vi "FSM.vi"() -> ()   [LabVIEW 2016]
doc: "Use this template to build a simple state machine design pattern. Each state executes code and determines which state to transition to."
uses:
  controls/State.ctl
panel:
  out "Long":bool
  in  "stop":bool
  in  "input1":bool
  in  "input 0":bool
  out "Select Sentence":bool
  out "Word Outputs":string[](array[string])=["", "", "", "", "", "", "", "h", "i", "j", "k", "l", "m", "n", "o", "p", "q", "r", "s", "t", "u", "v", "w", "x", "y", "z"]
  out "Length counter":i32
  out "Input RMS":dbl
  out "Slide":T1 scale=0.0..100.0
  in  "Dictionary Path":path
  out "DIGITS":string
  out "Letters Output":string
  in  "sentence2":string
  in  "sentence1":string
  in  "停止按钮":bool
  out "one":bool
  out "zero":bool
  in  "RMS threshold":dbl
  in  "Length threshold":i32=20
  in  "Input Gain":dbl
  out "Frequency response":dynamicdata(graph)
  out "Short":bool
  in  "Input TEST":dbl(slide) scale=0.0..10.0
  out "数组":string[](array[string])
  out "testforlin":string
  out "三位数":i32
  out "count digit":i32
  out "check code":bool
  out "Digits 2":bool[](array[boolean])
  out "index word mode":dbl
  out "add 0 （word mode）":bool
  out "counter2":dbl
  out "counter":dbl
  out "word index":dbl
  out "compare word":string
  out "Final Output":string
  out "instructions":string[](array[string])=["Hello", "Run", "Phone", "Cat", "Speak", "Mango", "Late", "EMG", "Volleyball", "Sing", "Over", "Maybe", "After", "Banana", "Love", "Sleep", "Too", "Hope", "Tomorrow", "Smile"]
  out "Last selected letter":string
  out "letters output (array)":string[](array[string])
  out "Current letter index":dbl
  out "Digits":bool[](array[boolean])
  out "Current digit index":dbl
  out "letter database":string[](array[string])=["Hello", "Run", "Phone", "Cat", "Speak", "Mango", "Late", "EMG", "Volleyball", "Sing", "Over", "Maybe", "After", "Banana", "Love", "Sleep", "Too", "Hope", "Tomorrow", "Smile"]
  out "Current state":T2=enum."Count digits"
  in  "Exit":bool
  # "Instruction Code:"
  # "Suggesting\nList"
  # "10000    p\n10001    q\n10010    r\n10011    s\n10100    t\n10101    u\n10110    v\n10111    w\n11000    x\n11001    y\n11010    z\n11011    clear letter\n11100    clear sentence\n\n11101    enter sentence 1\n\n\n11110    enter sentence 2\n\n11111    select word"
  # "00000    enter\n00001    a\n00010    b\n00011    c\n00100    d\n00101    e\n00110    f\n00111    g\n01000    h\n01001    i\n01010    j\n01011    k\n01100    l\n01101    m\n01110    n\n01111    o"
  # "TESTING"
  # "Input Parameters"
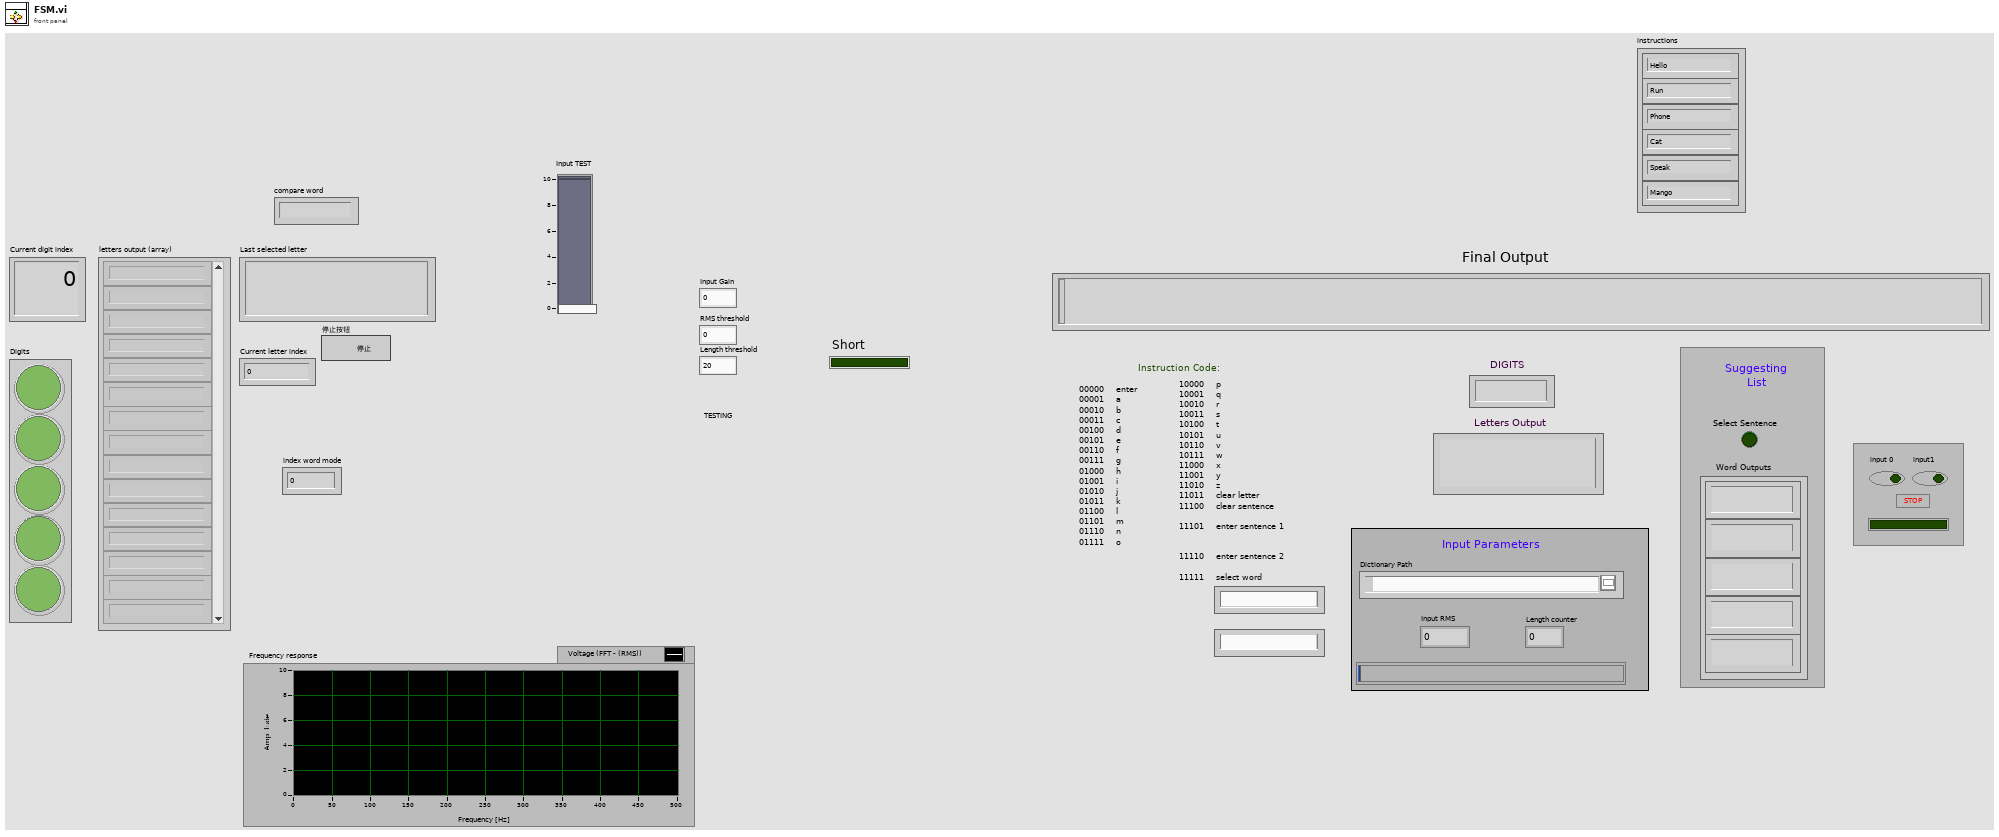
[diagram p1: front panel]
types:
  T1 = typedef "控件 1.ctl" = u8
  T2 = typedef "State.ctl" = enum16{"check code for word", "count digit for word", "add 1 word", "add 0 word", "pick word", "enter sentence3", "enter sentence2", "enter sentence1", "clear sentence", "enter word", "clear all", "check code", "Count digits", "Input signal", "Add digit 0", "Add digit 1", "Select word", "Reset digits", "Delete word", "Exit"}
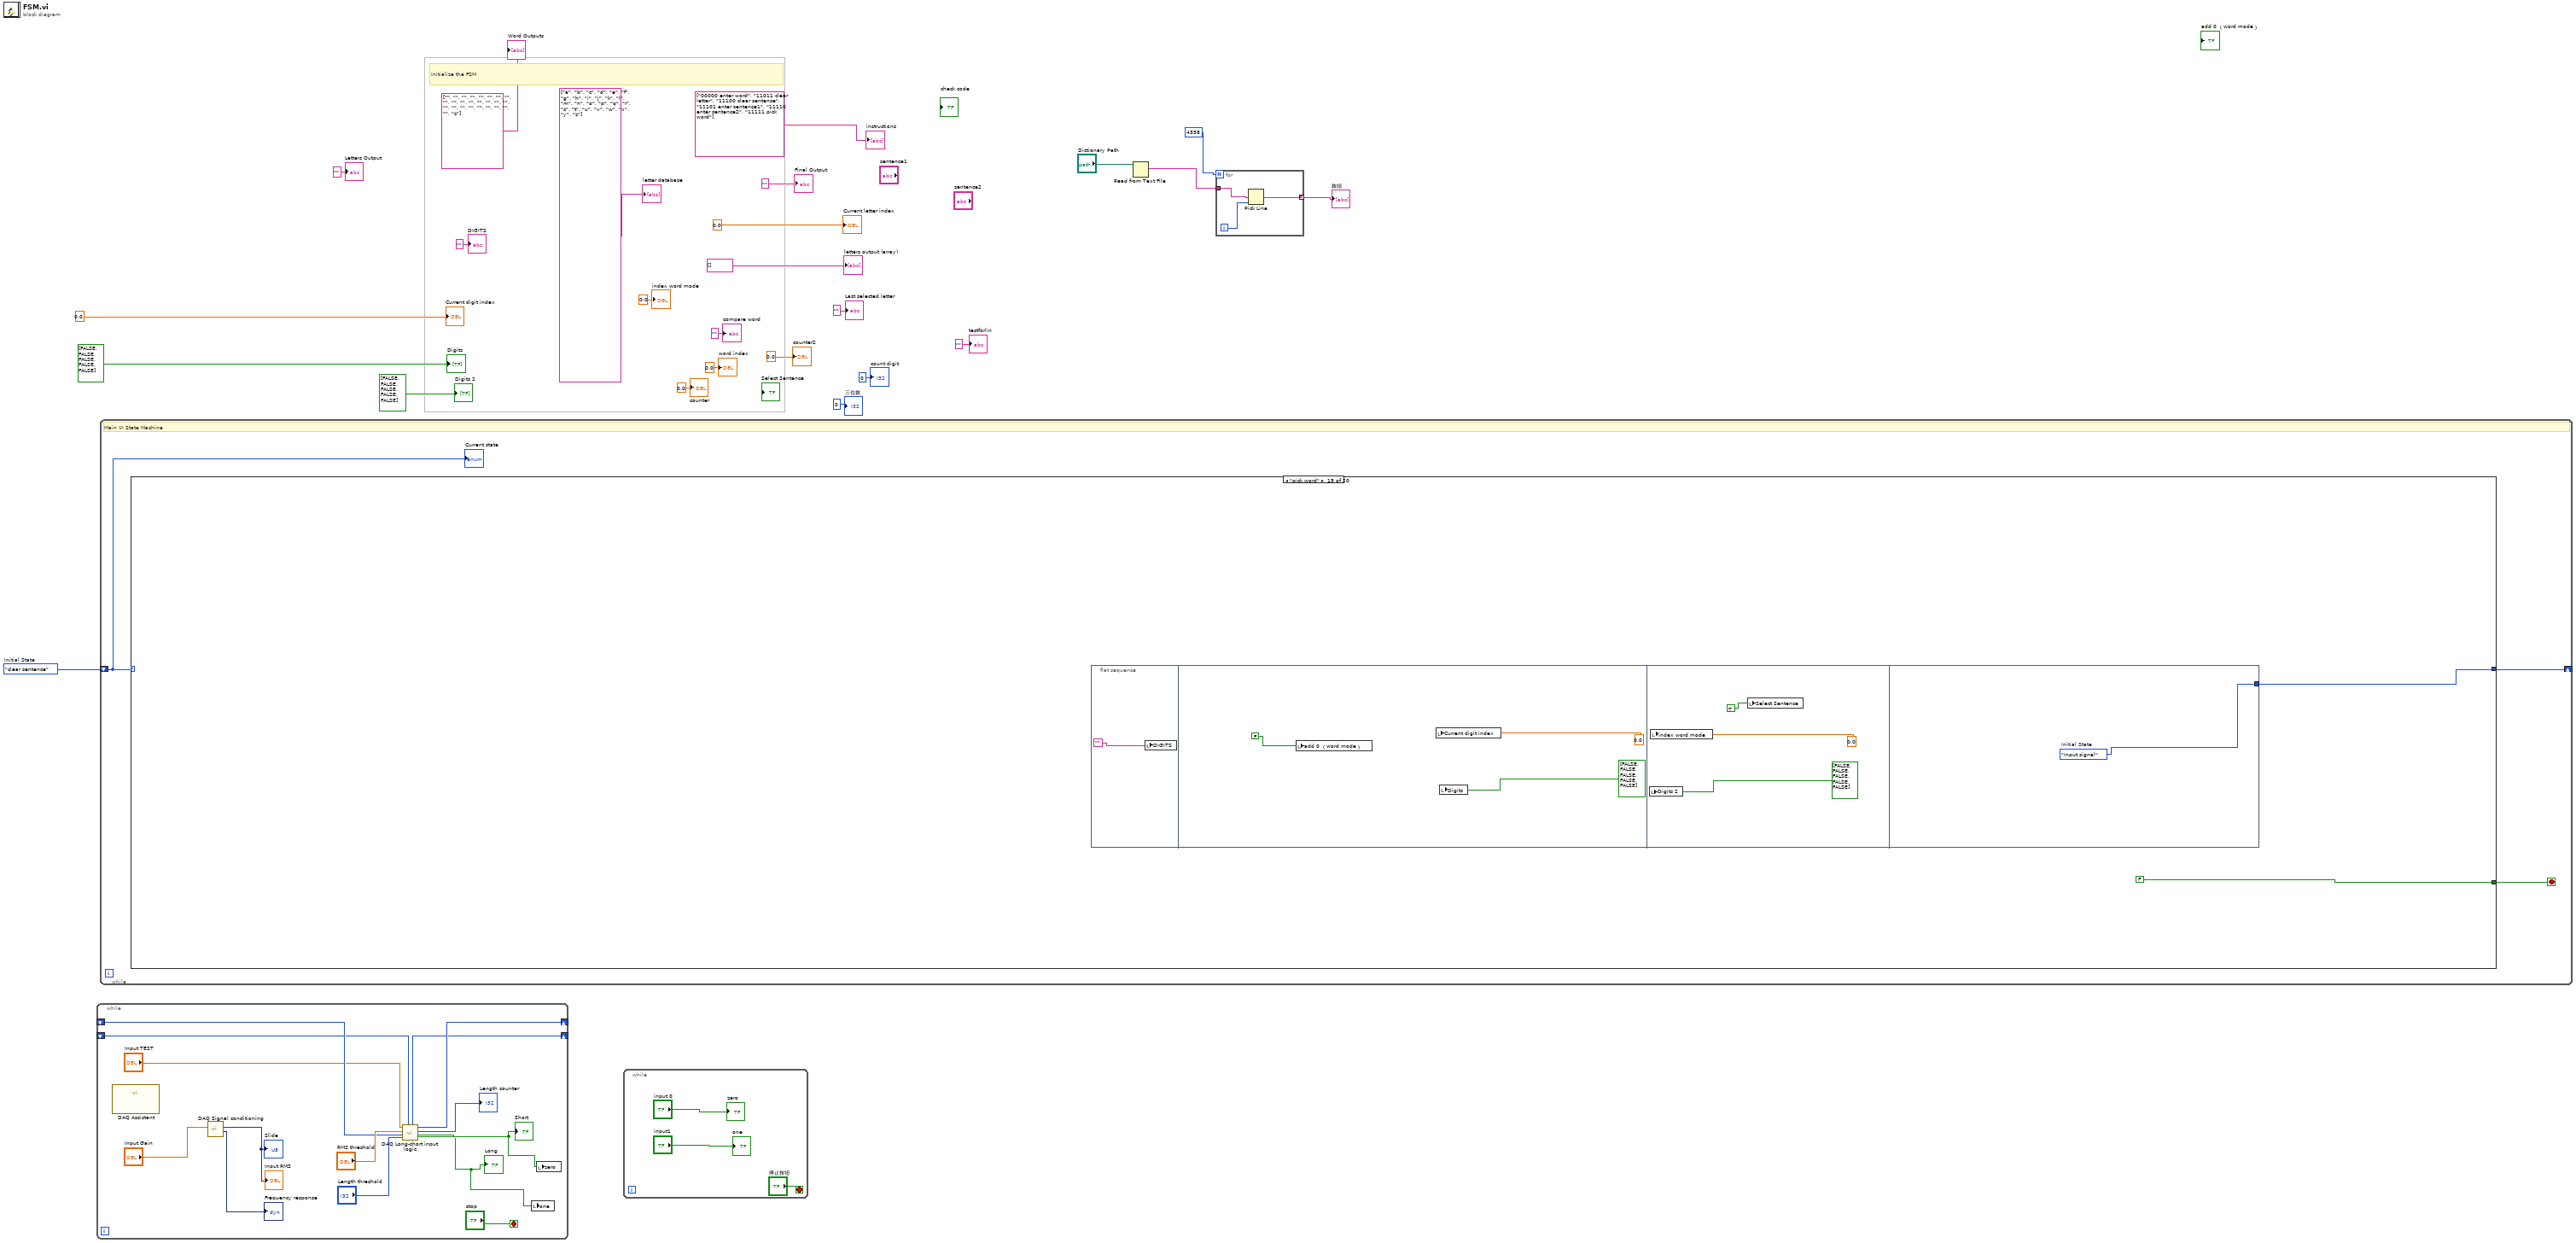
[diagram p0: block diagram]
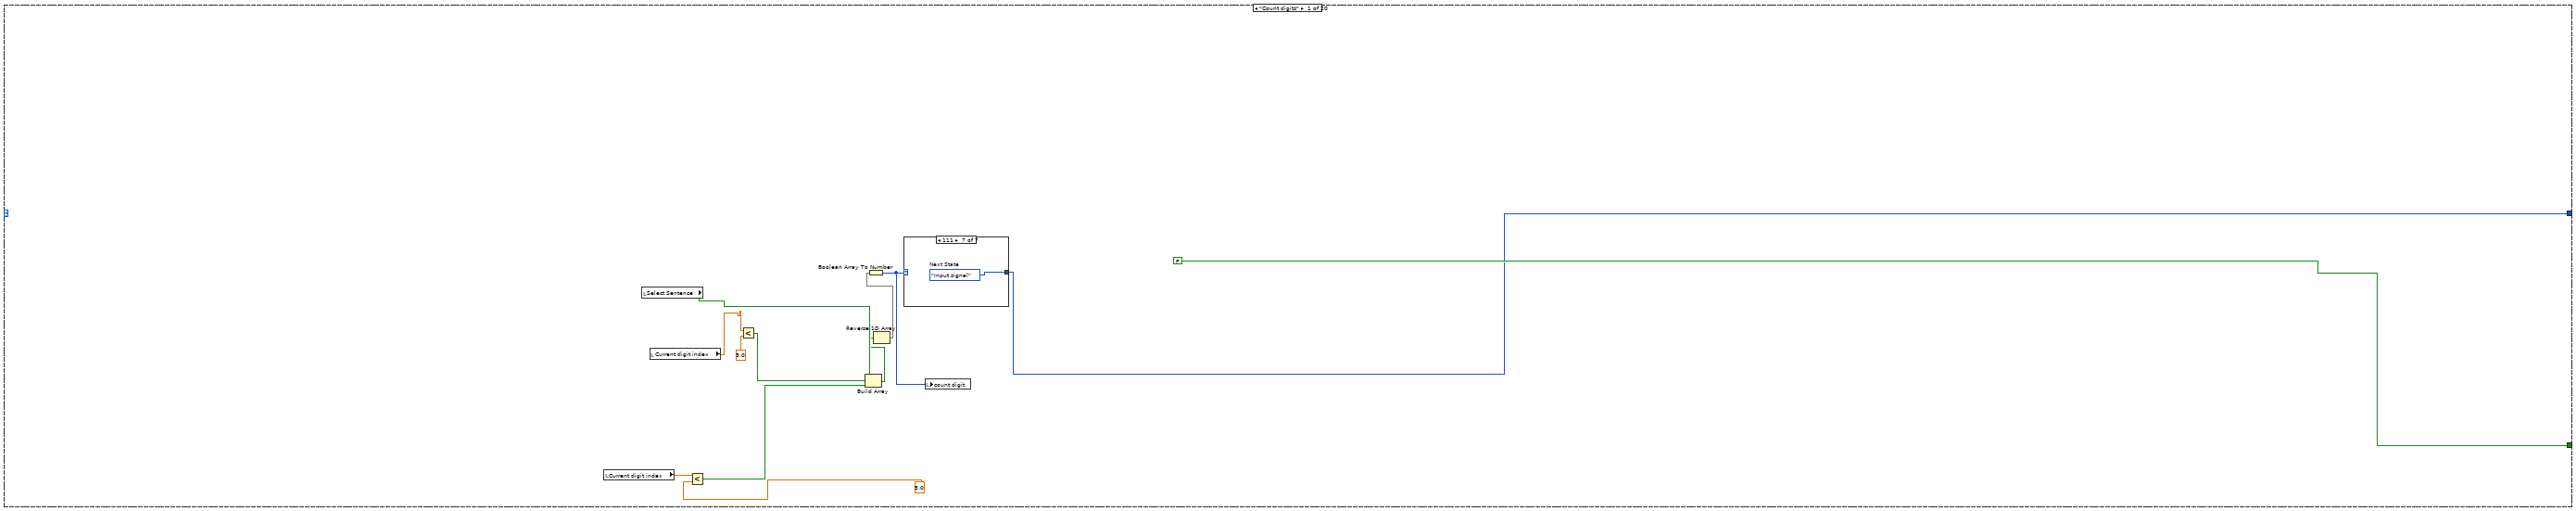
[diagram p2: hidden frame]
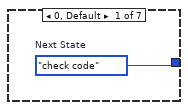
[diagram p3: hidden frame]
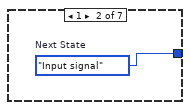
[diagram p4: hidden frame]
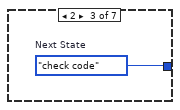
[diagram p5: hidden frame]
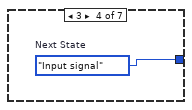
[diagram p6: hidden frame]
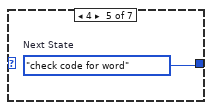
[diagram p7: hidden frame]
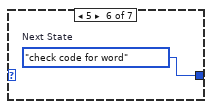
[diagram p8: hidden frame]
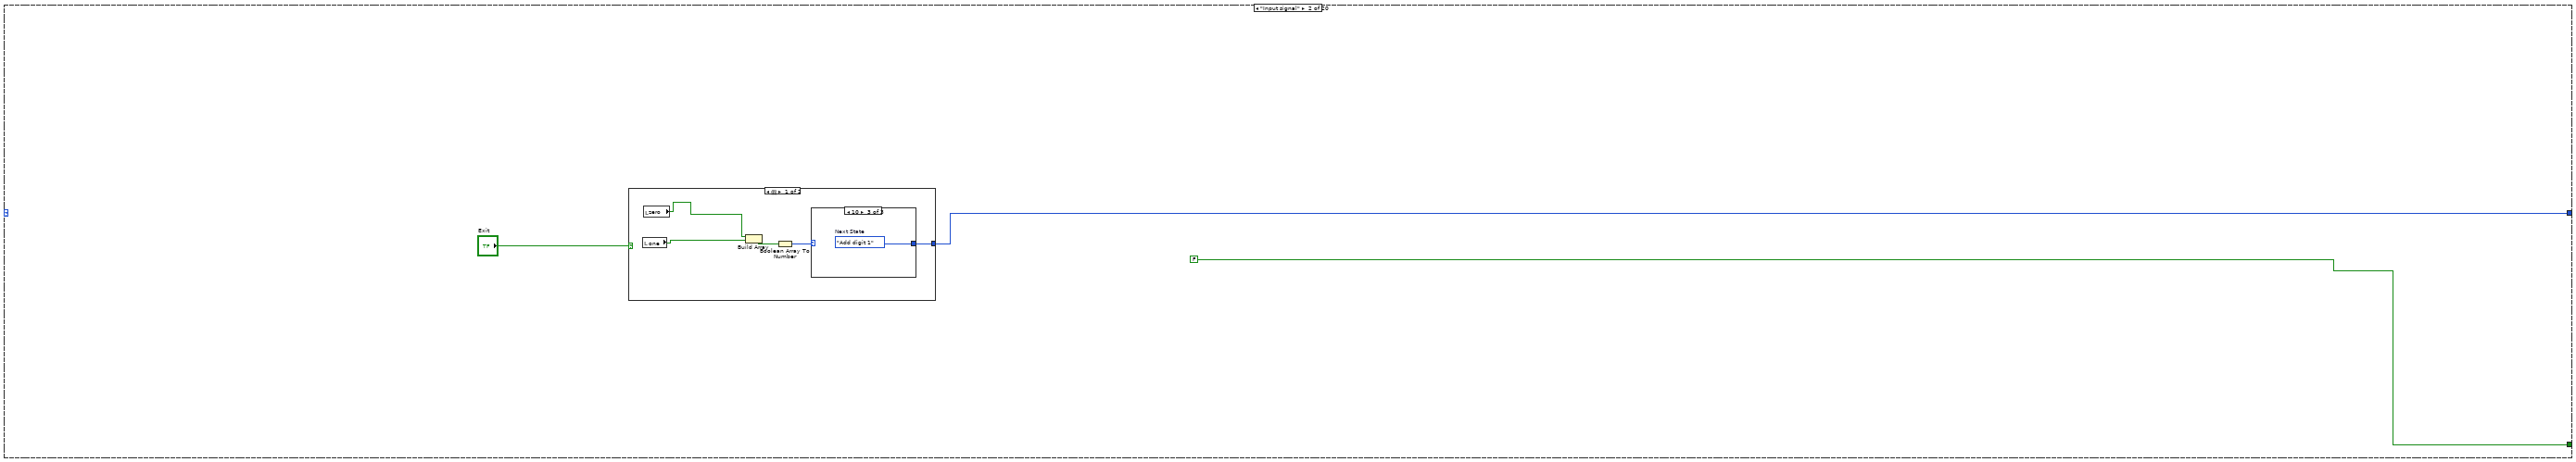
[diagram p9: hidden frame]
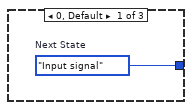
[diagram p10: hidden frame]
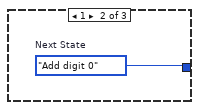
[diagram p11: hidden frame]
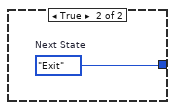
[diagram p12: hidden frame]
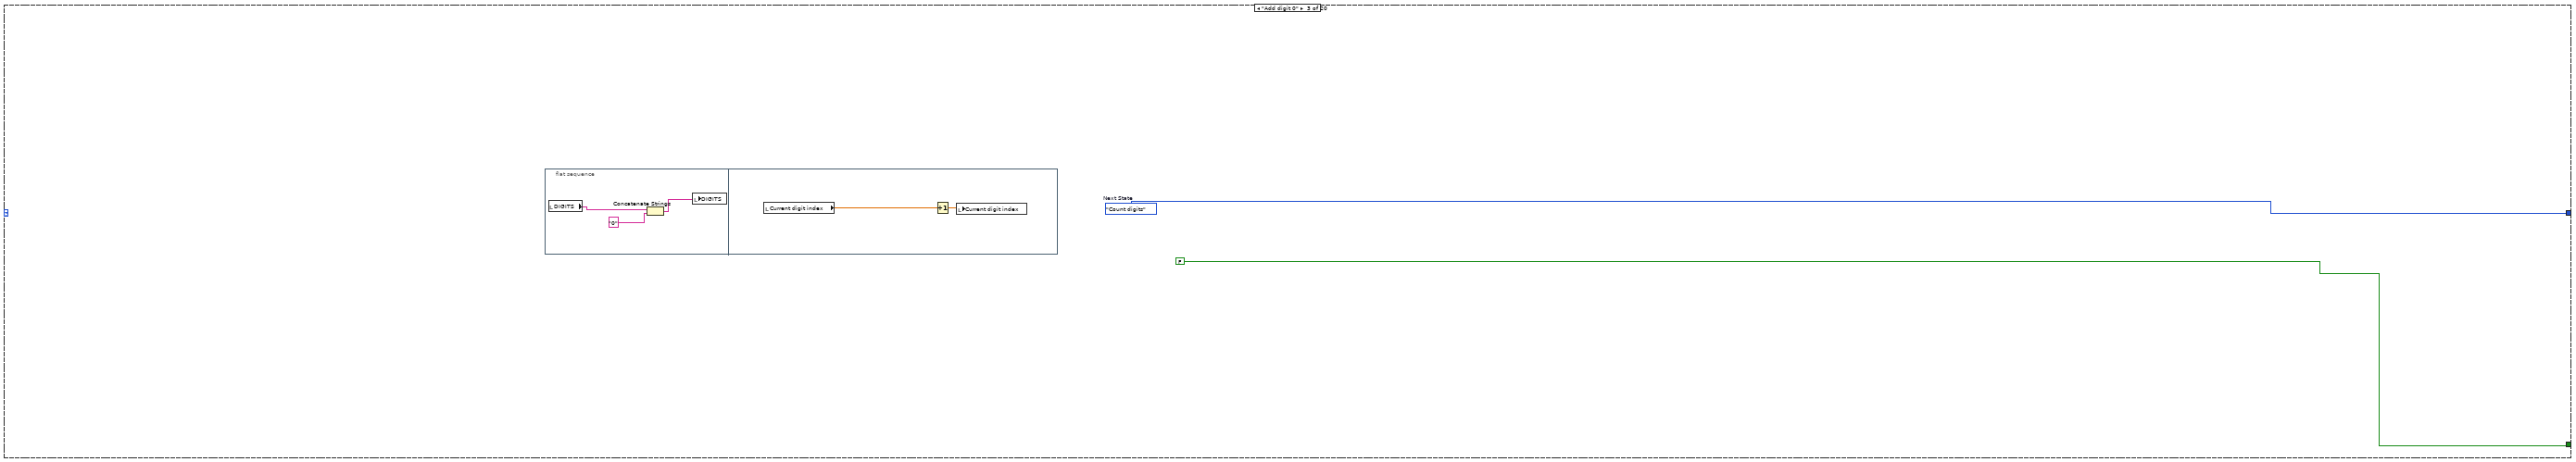
[diagram p13: hidden frame]
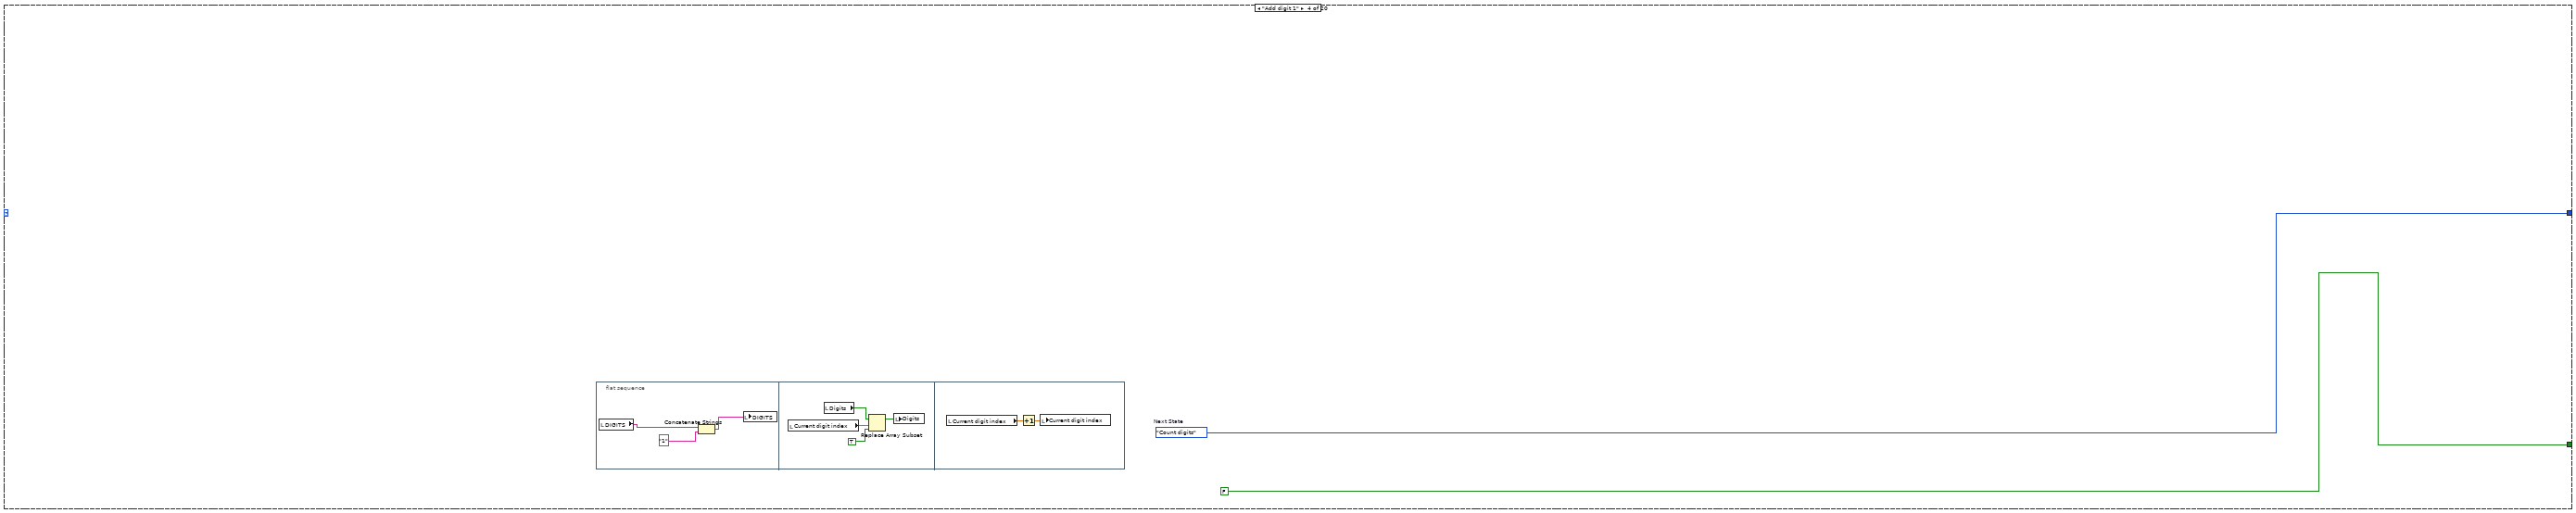
[diagram p14: hidden frame]
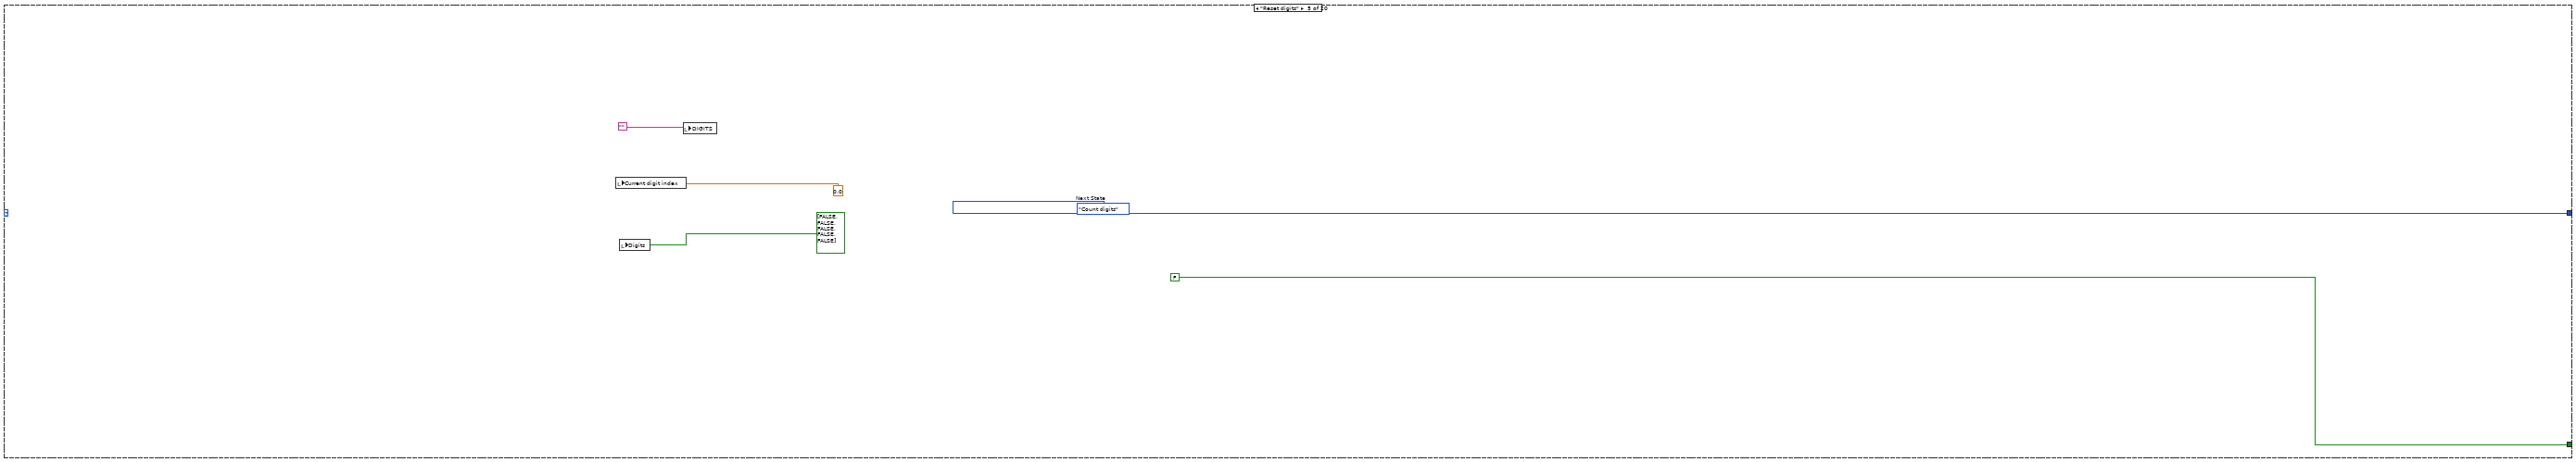
[diagram p15: hidden frame]
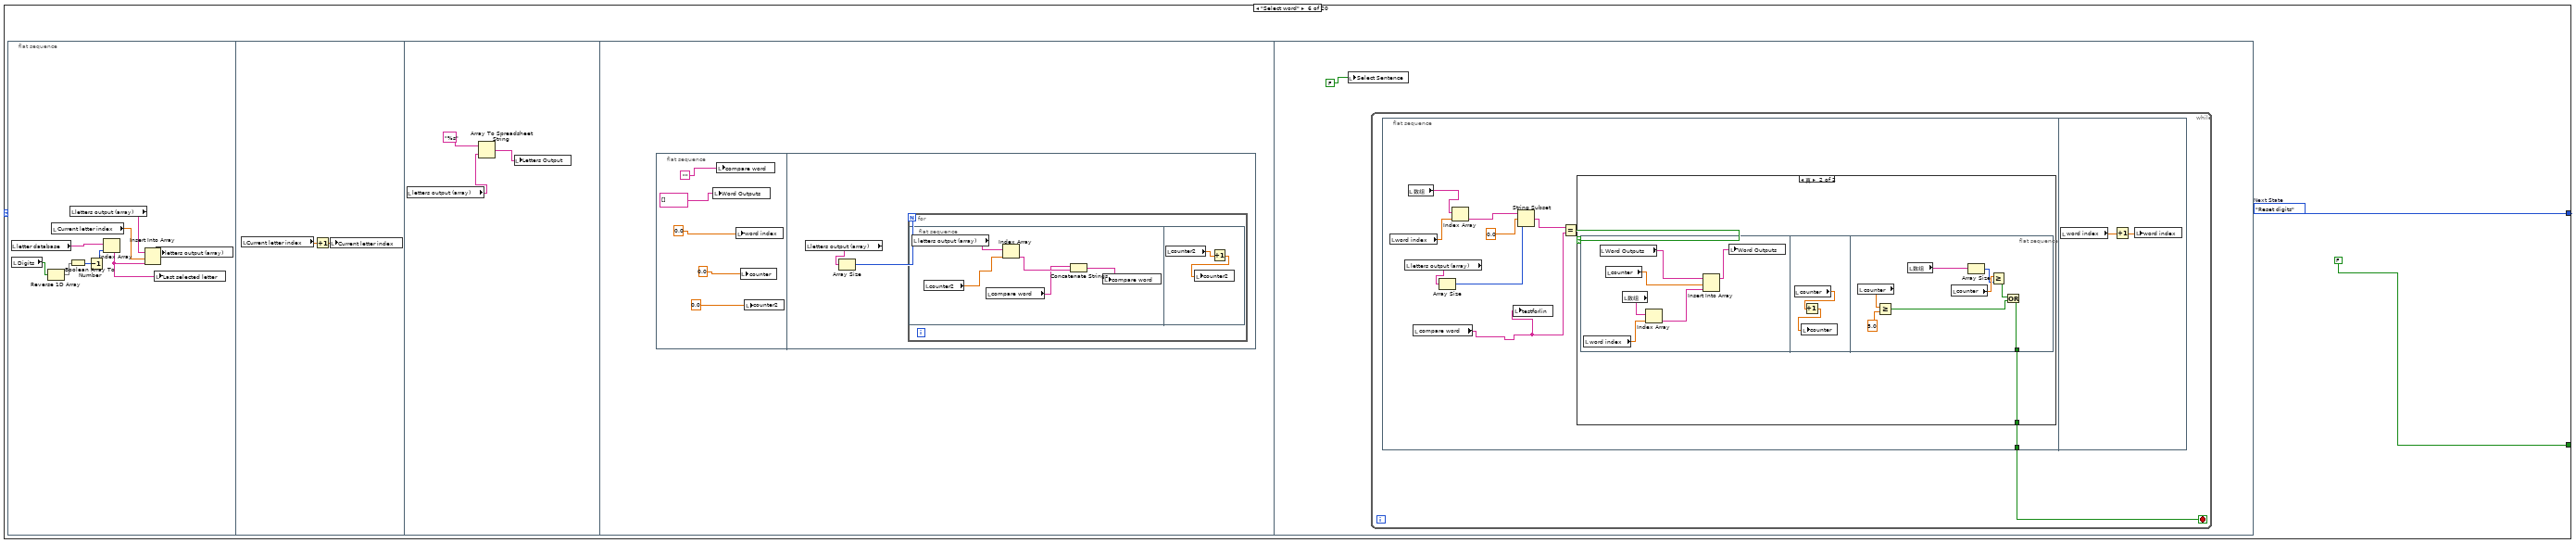
[diagram p16: hidden frame]
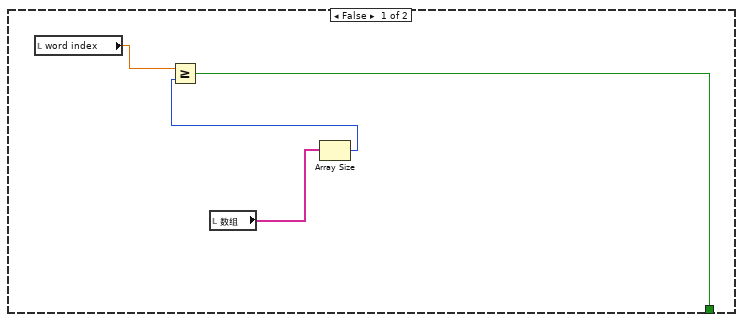
[diagram p17: hidden frame]
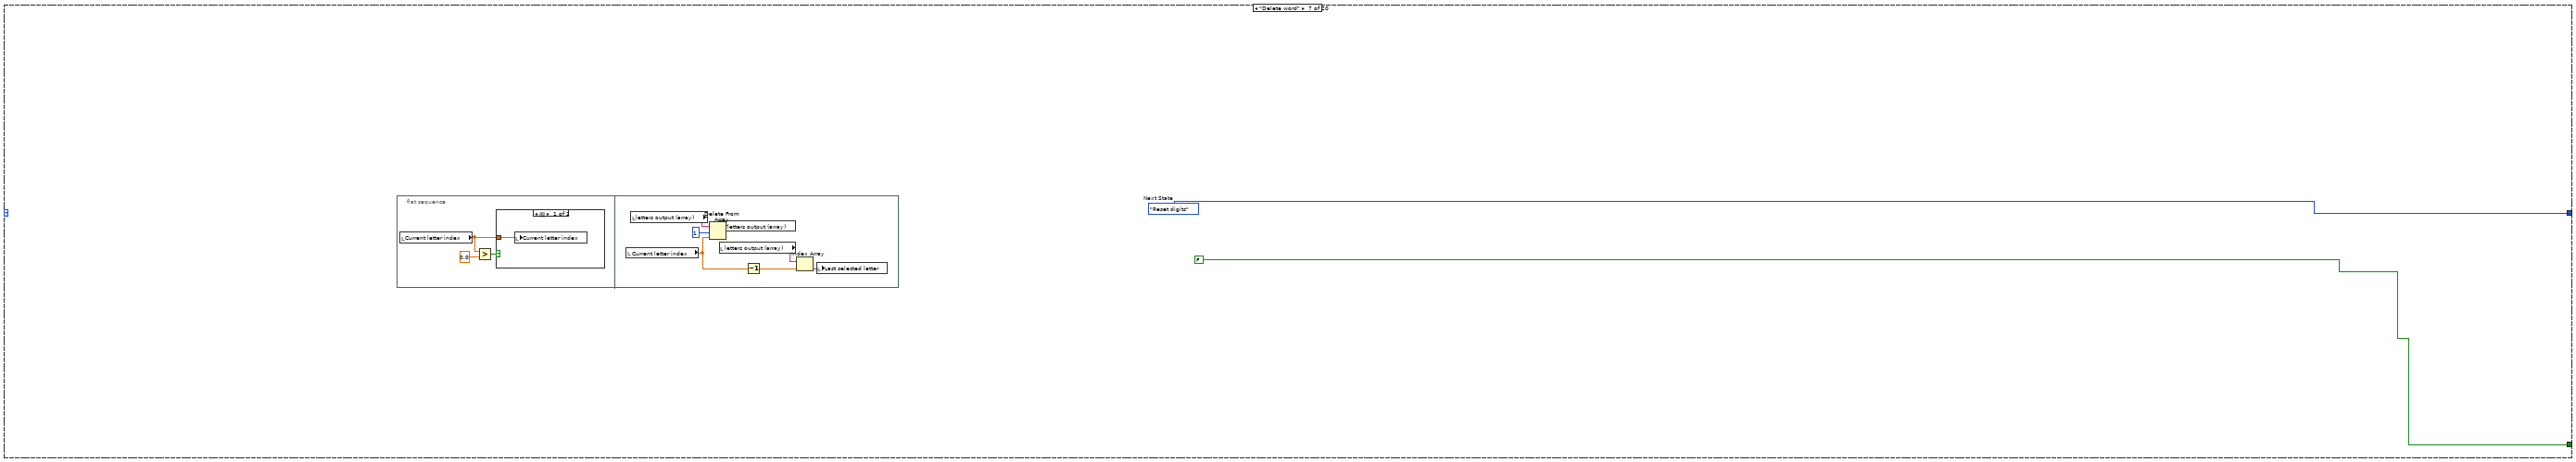
[diagram p18: hidden frame]
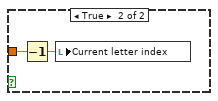
[diagram p19: hidden frame]
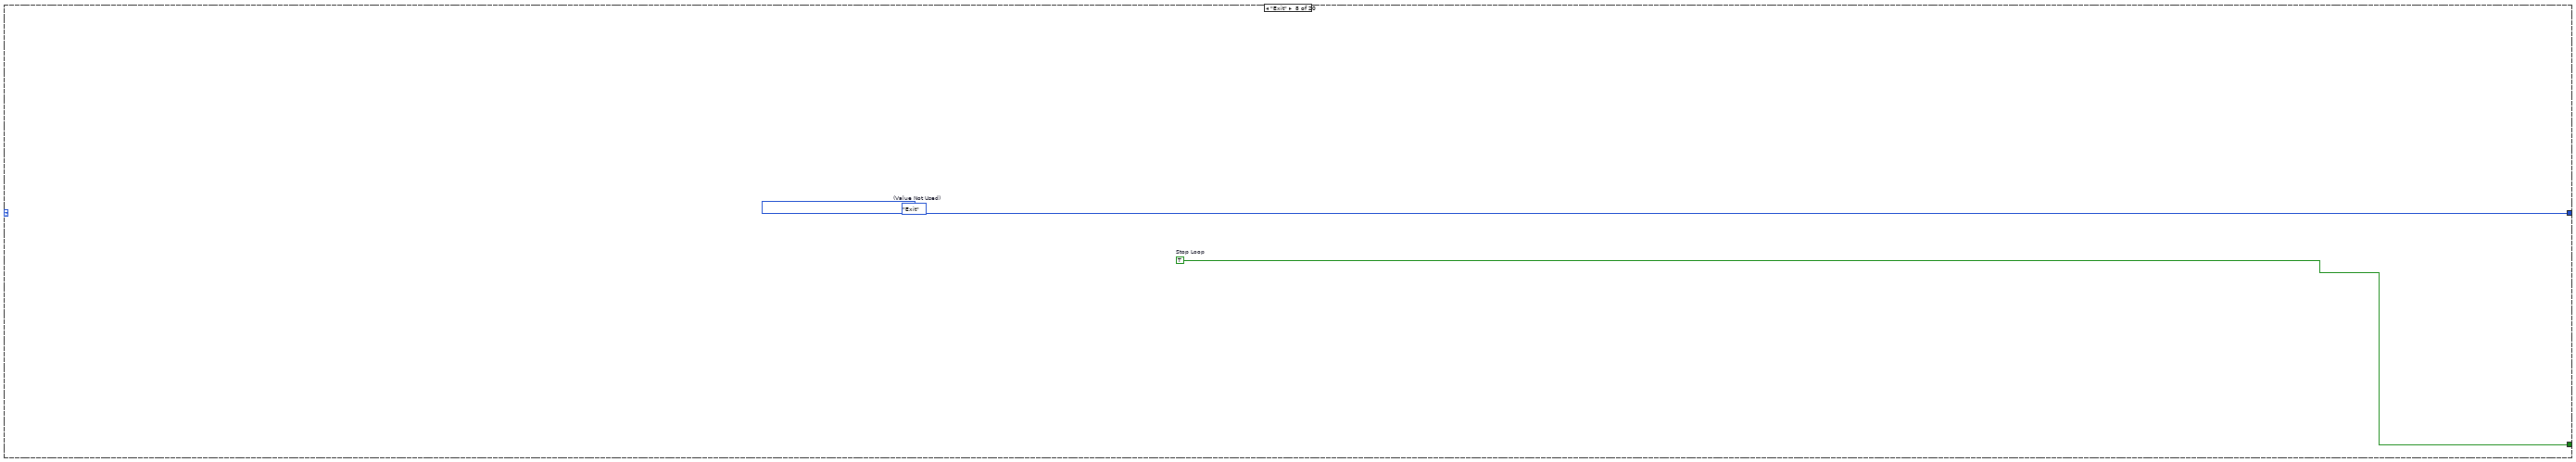
[diagram p20: hidden frame]
diagram:
  w25 = State."clear sentence"  # Initial State
  # "Initialize the FSM"
  n1 = while {
    shift-right: [w37] -> _
    shift-left: _ -> [w36]
    shift-right: [w34] -> _
    shift-left: _ -> [w35]
    stop <- "stop" stop-if-true
    n2 = call "DAQ Assistant"() -> ()  [unwired: 12 in]
    n3 = call "DAQ Signal conditioning.vi"("Gain"="Input Gain") -> ("FFT - (RMS)"=→"Frequency response":dynamicdata, "Dynamic Data"=→"Input RMS" →"Slide":dynamicdata)  [unwired: 9 in]
    n4 = call "DAQ Long-short input logic.vi"("Signal Length"="Length threshold", "Numeric in"=w35, "Numeric 3"=w36, "Threshold"="RMS threshold", "data"="Input TEST") -> ("Boolean"=w27:bool, "x+y"=→"Length counter":i32, "Numeric 4"=w37:i32, "Boolean 2"=w26:bool, "Numeric out"=w34:i32)  [unwired: 2 in]
    "Short" <- w27
    "Long" <- w26
    n5 = local write "one"(w26) -> ()
    n6 = local write "zero"(w27) -> ()
  }
  n7 = while {
    shift-right: [w41] -> _
    shift-left: w25 -> [w42]
    stop <- w40 stop-if-true
    # "Main VI State Machine"
    n8 = case "条件结构" shown="\"pick word\"" w42 {
      tunnel: [w49 w64 w75 w82 w96 w98 w163 w178 w184 w202 w212 w227 w231 w236 w240 w244 w249 w257 w265 w275] -> w41
      tunnel: [FALSE FALSE FALSE FALSE FALSE FALSE ("Stop Loop?") FALSE ("Stop Loop?") w177 FALSE FALSE FALSE FALSE FALSE FALSE FALSE FALSE FALSE FALSE FALSE FALSE] -> w40
      frame "Count digits" {
        n9 = local read "Current digit index"() -> (w52:dbl)
        n10 = local read "Select Sentence"() -> (w46:bool)
        n11 = local read "Current digit index"() -> (w51:dbl)
        n12 = Less?(x=w52, y=5.0) -> (x < y?=w45:bool)
        n13 = Less?(x=w51, y=3.0) -> (x < y?=w48:bool)
        n14 = Build Array(w46, w48, w45) -> (w43:bool[])
        n15 = Reverse 1D Array(array=w43) -> (reversed array=w44:bool[])
        n16 = Boolean Array To Number(Boolean array=w44) -> (number=w47:u32)
        n17 = case shown="111" w47 {
          tunnel: [w55 w56 w57 w58 w59 w60 w61] -> w49
          frame 0, Default {
            w55 = State."check code"  # Next State
          }
          frame 1 {
            w56 = State."Input signal"  # Next State
          }
          frame 2 {
            w57 = State."check code"  # Next State
          }
          frame 3 {
            w58 = State."Input signal"  # Next State
          }
          frame 4 {
            w59 = State."check code for word"  # Next State
          }
          frame 5 {
            w60 = State."check code for word"  # Next State
          }
          frame 7 {
            w61 = State."Input signal"  # Next State
          }
        }
        n18 = local write "count digit"(w47) -> ()
      }
      frame "Input signal" {
        n19 = case shown="假" "Exit" {
          tunnel: [w67 w73] -> w64
          frame False {
            n20 = local read "one"() -> (w65:bool)
            n21 = local read "zero"() -> (w66:bool)
            n22 = Build Array(w66, w65) -> (w69:bool[])
            n23 = Boolean Array To Number(Boolean array=w69) -> (number=w68:u32)
            n24 = case shown="10" w68 {
              tunnel: [w70 w71 w72] -> w67
              frame 0, Default {
                w70 = State."Input signal"  # Next State
              }
              frame 1 {
                w71 = State."Add digit 0"  # Next State
              }
              frame 2 {
                w72 = State."Add digit 1"  # Next State
              }
            }
          }
          frame True {
            w73 = State."Exit"  # Next State
          }
        }
      }
      frame "Add digit 0" {
        w75 = State."Count digits"  # Next State
        n25 = flat-sequence {
          frame #0 {
            n26 = local read "DIGITS"() -> (w76:string)
            n27 = Concatenate Strings(w76, "0") -> (w78:string)
            n28 = local write "DIGITS"(w78) -> ()
          }
          frame #1 {
            n29 = local read "Current digit index"() -> (w80:dbl)
            n30 = Increment(x=w80) -> (x+1=w79:dbl)
            n31 = local write "Current digit index"(w79) -> ()
          }
        }
      }
      frame "Add digit 1" {
        w82 = State."Count digits"  # Next State
        n32 = flat-sequence {
          frame #0 {
            n33 = local read "DIGITS"() -> (w85:string)
            n34 = Concatenate Strings(w85, "1") -> (w83:string)
            n35 = local write "DIGITS"(w83) -> ()
          }
          frame #1 {
            n36 = local read "Current digit index"() -> (w89:dbl)
            n37 = local read "Digits"() -> (w87:bool[])
            n38 = Replace Array Subset(array=w87, new element=TRUE, index=w89) -> (w86:bool[])
            n39 = local write "Digits"(w86) -> ()
          }
          frame #2 {
            n40 = local read "Current digit index"() -> (w91:dbl)
            n41 = Increment(x=w91) -> (x+1=w90:dbl)
            n42 = local write "Current digit index"(w90) -> ()
          }
        }
      }
      frame "Reset digits" {
        w96 = State."Count digits"  # Next State
        n43 = local write "Current digit index"(0.0 ("Current digit index")) -> ()
        n44 = local write "Digits"(bool[] [FALSE, FALSE, FALSE, FALSE, FALSE]) -> ()
        n45 = local write "DIGITS"("") -> ()
      }
      frame "Select word" {
        w98 = State."Reset digits"  # Next State
        # "User State 1 - Replace this state with functionality for your own application."
        n46 = flat-sequence {
          frame #0 {
            n47 = local read "letter database"() -> (w104:string[])
            n48 = local read "Digits"() -> (w102:bool[])
            n49 = Reverse 1D Array(array=w102) -> (reversed array=w101:bool[])
            n50 = local read "Current letter index"() -> (w105:dbl)
            n51 = local read "letters output (array)"() -> (w106:string[])
            n52 = Boolean Array To Number(Boolean array=w101) -> (number=w100:u32)
            n53 = Decrement(x=w100) -> (x-1=w99:u32)
            n54 = Index Array(array=w104, index=w99) -> (element=w103:string)
            n55 = Insert Into Array(array=w106, index=w105, new element=w103) -> (w107:string[])
            n56 = local write "Last selected letter"(w103) -> ()
            n57 = local write "letters output (array)"(w107) -> ()
          }
          frame #1 {
            n58 = local read "Current letter index"() -> (w109:dbl)
            n59 = Increment(x=w109) -> (x+1=w108:dbl)
            n60 = local write "Current letter index"(w108) -> ()
          }
          frame #2 {
            n61 = local read "letters output (array)"() -> (w112:string[])
            n62 = Array To Spreadsheet String(array=w112, 3:"%s") -> (spreadsheet string=w110:string)  [unwired: 1 in]
            n63 = local write "Letters Output"(w110) -> ()
          }
          frame #3 {
            n64 = flat-sequence {
              frame #0 {
                n65 = local write "Word Outputs"(string[] []) -> ()
                n66 = local write "compare word"("") -> ()
                n67 = local write "word index"(0.0) -> ()
                n68 = local write "counter"(0.0) -> ()
                n69 = local write "counter2"(0.0) -> ()
              }
              frame #1 {
                n70 = local read "letters output (array)"() -> (w118:string[])
                n71 = Array Size(array=w118) -> (size(s)=w119:i32)
                n72 = for {
                  N: w119 -> [_]
                  n73 = flat-sequence {
                    frame #0 {
                      n74 = local read "letters output (array)"() -> (w123:string[])
                      n75 = local read "counter2"() -> (w120:dbl)
                      n76 = local read "compare word"() -> (w121:string)
                      n77 = Index Array(array=w123, index=w120) -> (element=w124:string)
                      n78 = Concatenate Strings(w121, w124) -> (w122:string)
                      n79 = local write "compare word"(w122) -> ()
                    }
                    frame #1 {
                      n80 = local read "counter2"() -> (w126:dbl)
                      n81 = Increment(x=w126) -> (x+1=w125:dbl)
                      n82 = local write "counter2"(w125) -> ()
                    }
                  }
                }
              }
            }
          }
          frame #4 {
            n83 = local write "Select Sentence"(FALSE) -> ()
            n84 = while {
              stop <- w128 stop-if-true
              n85 = flat-sequence {
                tunnel: [w131] -> w128
                frame #0 {
                  n86 = local read "word index"() -> (w137:dbl)
                  n87 = local read "letters output (array)"() -> (w138:string[])
                  n88 = local read "数组"() -> (w130:string[])
                  n89 = local read "compare word"() -> (w129:string)
                  n90 = Array Size(array=w138) -> (size(s)=w135:i32)
                  n91 = Index Array(array=w130, index=w137) -> (element=w134:string)
                  n92 = local write "testforlin"(w129) -> ()
                  n93 = String Subset(string=w134, offset (0)=0.0, length (rest)=w135) -> (substring=w133:string)
                  n94 = Equal?(x=w133, y=w129) -> (x = y?=w132:bool)
                  n95 = case shown="真" w132 {
                    tunnel: [w140 w143] -> w131
                    frame False {
                      n96 = local read "word index"() -> (w142:dbl)
                      n97 = local read "数组"() -> (w139:string[])
                      n98 = Array Size(array=w139) -> (size(s)=w141:i32)
                      n99 = Greater Or Equal?(x=w142, y=w141) -> (x >= y?=w140:bool)
                    }
                    frame True {
                      n100 = flat-sequence {
                        tunnel: [w152] -> w143
                        frame #0 {
                          n101 = local read "word index"() -> (w147:dbl)
                          n102 = local read "Word Outputs"() -> (w144:string[])
                          n103 = local read "counter"() -> (w145:dbl)
                          n104 = local read "数组"() -> (w146:string[])
                          n105 = Index Array(array=w146, index=w147) -> (element=w148:string)
                          n106 = Insert Into Array(array=w144, index=w145, new element=w148) -> (w149:string[])
                          n107 = local write "Word Outputs"(w149) -> ()
                        }
                        frame #1 {
                          n108 = local read "counter"() -> (w151:dbl)
                          n109 = Increment(x=w151) -> (x+1=w150:dbl)
                          n110 = local write "counter"(w150) -> ()
                        }
                        frame #2 {
                          n111 = local read "counter"() -> (w158:dbl)
                          n112 = Greater Or Equal?(x=w158, y=5.0) -> (x >= y?=w156:bool)
                          n113 = local read "数组"() -> (w157:string[])
                          n114 = local read "counter"() -> (w154:dbl)
                          n115 = Array Size(array=w157) -> (size(s)=w153:i32)
                          n116 = Greater Or Equal?(x=w154, y=w153) -> (x >= y?=w155:bool)
                          n117 = Or(x=w155, y=w156) -> (x .or. y?=w152:bool)
                        }
                      }
                    }
                  }
                }
                frame #1 {
                  n118 = local read "word index"() -> (w160:dbl)
                  n119 = Increment(x=w160) -> (x+1=w161:dbl)
                  n120 = local write "word index"(w161) -> ()
                }
              }
            }
          }
        }
      }
      frame "Delete word" {
        w163 = State."Reset digits"  # Next State
        n121 = flat-sequence {
          frame #0 {
            n122 = local read "Current letter index"() -> (w164:dbl)
            n123 = Greater?(x=w164, y=0.0) -> (0:w165:bool)
            n124 = case shown="假" w165 {
              tunnel: w164 -> [w167 w169]
              frame False {
                n125 = local write "Current letter index"(w167) -> ()
              }
              frame True {
                n126 = Decrement(x=w169) -> (x-1=w168:dbl)
                n127 = local write "Current letter index"(w168) -> ()
              }
            }
          }
          frame #1 {
            n128 = local read "Current letter index"() -> (w170:dbl)
            n129 = local read "letters output (array)"() -> (w176:string[])
            n130 = Delete From Array(array=w176, length=1, index=w170) -> (array with subset deleted=w174:string[])  [unwired: 1 out]
            n131 = local write "letters output (array)"(w174) -> ()
            n132 = local read "letters output (array)"() -> (w172:string[])
            n133 = Decrement(x=w170) -> (x-1=w173:dbl)
            n134 = Index Array(array=w172, index=w173) -> (element=w171:string)
            n135 = local write "Last selected letter"(w171) -> ()
          }
        }
      }
      frame "Exit" {
        w177 = TRUE  # Stop Loop
        w178 = State."Exit"  # (Value Not Used)
        # "Exit - Exit the application and stops the DAQ VI."
      }
      frame "check code" {
        n136 = local read "Digits"() -> (w183:bool[])
        n137 = Reverse 1D Array(array=w183) -> (reversed array=w182:bool[])
        n138 = Boolean Array To Number(Boolean array=w182) -> (number=w180:u32)
        n139 = Less Or Equal?(x=w180, y=26.0) -> (x <= y?=w187:bool)
        n140 = Greater Or Equal?(x=w180, y=1.0) -> (x >= y?=w186:bool)
        n141 = And(x=w187, y=w186) -> (x .and. y?=w185:bool)
        n142 = local write "check code"(FALSE) -> ()
        n143 = case shown="假" w185 {
          tunnel: [w191 State."Select word"] -> w184
          tunnel: w180 -> [w190 _]
          frame False {
            n144 = case shown="11110" w190 {
              tunnel: [w192 State."clear all" w194 w195 w196 w197] -> w191
              frame 0, Default {
                w192 = State."enter word"  # Next State
              }
              frame 27 {
              }
              frame 28 {
                w194 = State."clear sentence"  # Initial State
              }
              frame 29 {
                w195 = State."enter sentence1"  # Initial State
              }
              frame 30 {
                w196 = State."enter sentence2"  # Initial State
              }
              frame 31 {
                w197 = State."pick word"  # Initial State
              }
            }
          }
          frame True {
          }
        }
      }
      frame "clear all" {
        w202 = State."Count digits"  # Next State
        n145 = flat-sequence {
          frame #0 {
            n146 = local write "Current digit index"(0.0 ("Current digit index")) -> ()
            n147 = local write "Digits"(bool[] [FALSE, FALSE, FALSE, FALSE, FALSE]) -> ()
          }
          frame #1 {
            n148 = local write "Current letter index"(0.0) -> ()
          }
          frame #2 {
            n149 = local read "letters output (array)"() -> (w207:string[])
            n150 = Array Size(array=w207) -> (size(s)=w206:i32)
            n151 = for {
              N: w206 -> [_]
              n152 = local read "letters output (array)"() -> (w208:string[])
              n153 = Delete From Array(array=w208, length=1) -> (array with subset deleted=w209:string[])  [unwired: 1 in, 1 out]
              n154 = local write "letters output (array)"(w209) -> ()
            }
          }
        }
        n155 = local write "Select Sentence"(FALSE) -> ()
        n156 = local write "DIGITS"("") -> ()
      }
      frame "enter word" {
        w212 = State."clear all"  # Initial State
        n157 = flat-sequence {
          frame #0 {
            n158 = local write "Current letter index"(0.0) -> ()
          }
          frame #1 {
            n159 = local read "letters output (array)"() -> (w215:string[])
            n160 = Array Size(array=w215) -> (size(s)=w214:i32)
            n161 = for {
              N: w214 -> [_]
              n162 = flat-sequence {
                frame #0 {
                  n163 = local read "letters output (array)"() -> (w220:string[])
                  n164 = local read "Current letter index"() -> (w219:dbl)
                  n165 = Index Array(array=w220, index=w219) -> (element=w216:string)
                  n166 = local read "Final Output"() -> (w217:string)
                  n167 = Concatenate Strings(w217, w216) -> (w218:string)
                  n168 = local write "Final Output"(w218) -> ()
                }
                frame #1 {
                  n169 = local read "Current letter index"() -> (w222:dbl)
                  n170 = Increment(x=w222) -> (x+1=w221:dbl)
                  n171 = local write "Current letter index"(w221) -> ()
                }
              }
            }
          }
          frame #2 {
            n172 = local read "Final Output"() -> (w225:string)
            n173 = call <vilib>:"Space Constant.vi"() -> ("String"=w224:string)
            n174 = Concatenate Strings(w225, w224) -> (w223:string)
            n175 = local write "Final Output"(w223) -> ()
          }
        }
      }
      frame "clear sentence" {
        w227 = State."clear all"  # Initial State
        n176 = local write "Final Output"("") -> ()
      }
      frame "enter sentence1" {
        w231 = State."Reset digits"  # Initial State
        n177 = local read "sentence1"() -> (w229:string)
        n178 = Concatenate Strings("", w229) -> (w232:string)
        n179 = local write "Final Output"(w232) -> ()
      }
      frame "enter sentence2" {
        w236 = State."Reset digits"  # Initial State
        n180 = local read "sentence2"() -> (w234:string)
        n181 = Concatenate Strings("", w234) -> (w237:string)
        n182 = local write "Final Output"(w237) -> ()
      }
      frame "enter sentence3" {
        w240 = State."Reset digits"  # Initial State
        n183 = Concatenate Strings("", "time to take medicine") -> (w241:string)
        n184 = local write "Final Output"(w241) -> ()
      }
      frame "add 0 word" {
        w244 = State."count digit for word"  # Next State
        n185 = flat-sequence {
          frame #0 {
            n186 = local write "add 0 （word mode）"(TRUE) -> ()
          }
          frame #1 {
            n187 = local read "index word mode"() -> (w248:dbl)
            n188 = Increment(x=w248) -> (x+1=w247:dbl)
            n189 = local write "index word mode"(w247) -> ()
          }
        }
      }
      frame "add 1 word" {
        w249 = State."count digit for word"  # Next State
        n190 = flat-sequence {
          frame #0 {
            n191 = local read "index word mode"() -> (w254:dbl)
            n192 = local read "Digits 2"() -> (w252:bool[])
            n193 = Replace Array Subset(array=w252, new element=TRUE, index=w254) -> (w251:bool[])
            n194 = local write "Digits"(w251) -> ()
          }
          frame #1 {
            n195 = local read "index word mode"() -> (w256:dbl)
            n196 = Increment(x=w256) -> (x+1=w255:dbl)
            n197 = local write "index word mode"(w255) -> ()
          }
        }
      }
      frame "count digit for word" {
        n198 = local read "index word mode"() -> (w259:dbl)
        n199 = Less?(x=w259, y=3.0) -> (x < y?=w260:bool)
        n200 = case shown="假" w260 {
          tunnel: [w262 w263] -> w257
          frame False {
            w262 = State."check code for word"  # Next State
          }
          frame True {
            w263 = State."pick word"  # Next State
          }
        }
      }
      frame "pick word" {
        n201 = flat-sequence {
          tunnel: [w273] -> w265
          frame #0 {
            n202 = local write "DIGITS"("") -> ()
          }
          frame #1 {
            n203 = local write "add 0 （word mode）"(FALSE) -> ()
            n204 = local write "Current digit index"(0.0 ("Current digit index")) -> ()
            n205 = local write "Digits"(bool[] [FALSE, FALSE, FALSE, FALSE, FALSE]) -> ()
          }
          frame #2 {
            n206 = local write "Digits 2"(bool[] [FALSE, FALSE, FALSE, FALSE, FALSE]) -> ()
            n207 = local write "index word mode"(0.0 ("Current digit index")) -> ()
            n208 = local write "Select Sentence"(TRUE) -> ()
          }
          frame #3 {
            w273 = State."Input signal"  # Initial State
          }
        }
      }
      frame "check code for word" {
        w275 = State."clear all"  # Initial State
        n209 = flat-sequence {
          frame #0 {
            n210 = local write "DIGITS"("") -> ()
          }
          frame #1 {
            n211 = local read "Digits"() -> (w287:bool[])
            n212 = local read "Word Outputs"() -> (w285:string[])
            n213 = Reverse 1D Array(array=w287) -> (reversed array=w286:bool[])
            n214 = Boolean Array To Number(Boolean array=w286) -> (number=w282:u32)
            n215 = local read "Final Output"() -> (w284:string)
            n216 = Divide(x=w282, y=4) -> (x/y=w277:dbl)
            n217 = local write "三位数"(w277) -> ()
            n218 = Index Array(array=w285, index=w277) -> (element=w283:string)
            n219 = Concatenate Strings(w284, w283) -> (w280:string)
            n220 = call <vilib>:"Space Constant.vi"() -> ("String"=w279:string)
            n221 = Concatenate Strings(w280, w279) -> (w278:string)
            n222 = local write "Final Output"(w278) -> ()
          }
        }
      }
    }
    "Current state" <- w42
  }
  n223 = while {
    stop <- "停止按钮" stop-if-true
    "zero" <- "input 0"
    "one" <- "input1"
  }
  n224 = Read from Text File(file (use dialog)="Dictionary Path") -> (text=w6:string)  [unwired: 3 in, 3 out]
  n225 = for {
    N: 4338 -> [_]
    tunnel: w6 -> [w293]
    tunnel: [w292] -> w5 mode=indexing
    i -> [w291]
    n226 = Pick Line(multi-line string=w293, line index=w291) -> (output string=w292:string)  [unwired: 1 in]
  }
  "数组" <- w5
  "letter database" <- string[] ["a", "b", "c", "d", "e", "f", "g", "h", "i", "j", "k", "l", "m", "n", "o", "p", "q", "r", "s", "t", "u", "v", "w", "x", "y", "z"] ("Word database")
  "Current digit index" <- 0.0 ("Current digit index")
  "Digits" <- bool[] [FALSE, FALSE, FALSE, FALSE, FALSE]
  "Current letter index" <- 0.0 ("Current digit index")
  "letters output (array)" <- string[] [] ("Words output")
  "Last selected letter" <- "" ("Last selected word")
  "instructions" <- string[] ["00000 enter word", "11011 clear letter", "11100 clear sentence", "11101 enter sentence1", "11110 enter sentence2", "11111 pick word"] ("Word database")
  "Final Output" <- ""
  "compare word" <- ""
  "word index" <- 0.0
  "Word Outputs" <- string[] ["", "", "", "", "", "", "", "", "", "", "", "", "", "", "", "", "", "", "", "", "", "", "", "", "", "z"] ("Word database")
  "counter" <- 0.0
  "counter2" <- 0.0
  "index word mode" <- 0.0
  "Digits 2" <- bool[] [FALSE, FALSE, FALSE, FALSE, FALSE]
  "count digit" <- 0
  "三位数" <- 0
  "testforlin" <- ""
  "Letters Output" <- ""
  "DIGITS" <- ""
